vi "Sets the ramp time for MANU.vi"(5 "Enable to Query":bool, 7 "Enable to Setup":bool, 8 "error in":errorcluster, 10 "Ramp Time":sgl=0.1 min=0.1 max=999.9 format="%.1f", 11 "VISA resource name":refnum<visa-resource-name>) -> (0 "error out":errorcluster, 2 "Return the Ramp Time":string, 3 "VISA resource name out":refnum<visa-resource-name>)   [LabVIEW 2021, in "GPT-9000.lvlib"]
uses:
  GPT-9000.lvlib
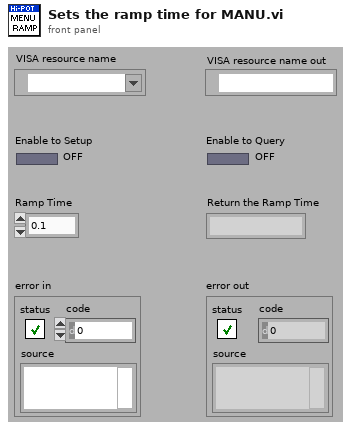
[diagram p1: front panel]
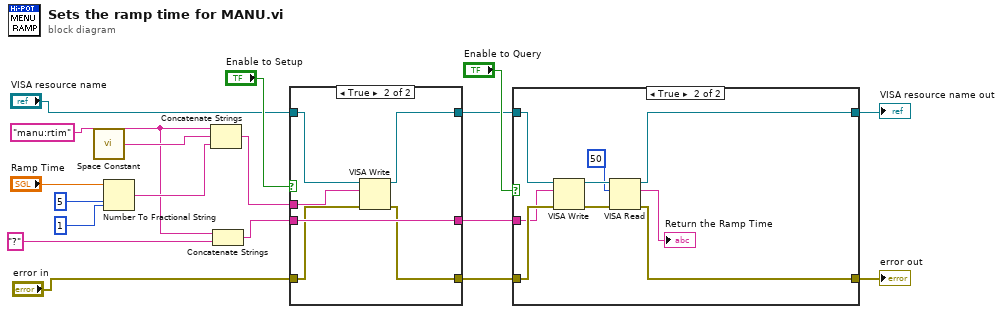
[diagram p0: block diagram]
diagram:
  w13 = "manu:rtim"
  n1 = call <vilib>:"Space Constant.vi"() -> ("String"=w16:string)
  n2 = Number To Fractional String(number="Ramp Time", width (-)=i16 5, precision (6)=i16 1) -> (F-format string=w15:string)  [unwired: 1 in]
  n3 = Concatenate Strings(w13, w16, w15) -> (w10:string)
  n4 = Concatenate Strings(w13, "?") -> (w9:string)
  n5 = case shown="True" "Enable to Setup" {
    tunnel: w10 -> [_ w22]
    tunnel: w9 -> [w19 w27]
    tunnel: "VISA resource name" -> [w21 w26]
    tunnel: "error in" -> [w20 w25]
    tunnel: [w21 w24] -> w5
    tunnel: [w20 w23] -> w4
    tunnel: [w19 w27] -> w3
    frame False {
    }
    frame True {
      n6 = VISA Write(VISA resource name=w26, write buffer=w22, error in (no error)=w25) -> (VISA resource name out=w24:refnum<visa-resource-name>, error out=w23:errorcluster)  [unwired: 1 out]
    }
  }
  n7 = case shown="True" "Enable to Query" {
    tunnel: w5 -> [w29 w36]
    tunnel: [w29 w32] -> w2
    tunnel: w4 -> [w28 w35]
    tunnel: [w28 w31] -> w1
    tunnel: w3 -> [_ w34]
    frame False {
    }
    frame True {
      n8 = VISA Write(VISA resource name=w36, write buffer=w34, error in (no error)=w35) -> (VISA resource name out=w37:refnum<visa-resource-name>, error out=w38:errorcluster)  [unwired: 1 out]
      n9 = VISA Read(VISA resource name=w37, byte count=u32 50, error in (no error)=w38) -> (VISA resource name out=w32:refnum<visa-resource-name>, read buffer=→"Return the Ramp Time":string, error out=w31:errorcluster)  [unwired: 1 out]
    }
  }
  "VISA resource name out" <- w2
  "error out" <- w1
